vi "Insert_SubPnl.vi"(0 "reference in":refnum<class "GUI.lvclass">, 1 "SubPnl":refnum<vi>, 11 "error in (no error)":errorcluster) -> (4 "reference out":refnum<class "GUI.lvclass">, 14 "dt":u32, 15 "error out":errorcluster)   [LabVIEW 2019, in "GUI.lvclass"]
uses:
  GUI.lvclass
  GUI.lvclass/GUI.ctl
  WindowsState.ctl
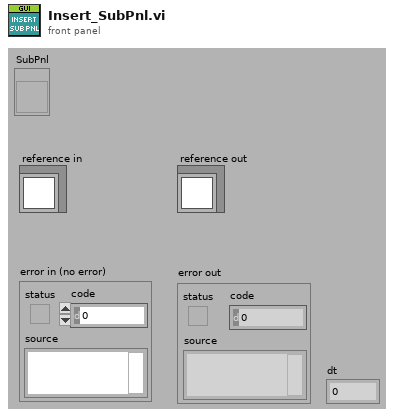
[diagram p1: front panel]
types:
  T1 = typedef "GUI.lvclass/WindowsState.ctl" = enum16{"NotReady", "Ready", "Inserted", "Opened"}
  T2 = typedef "GUI.lvclass/Shered Data.ctl" = cluster{"WindowsState":T1, "UI VI":refnum<vi>, "SubPnl":refnum<vi>}
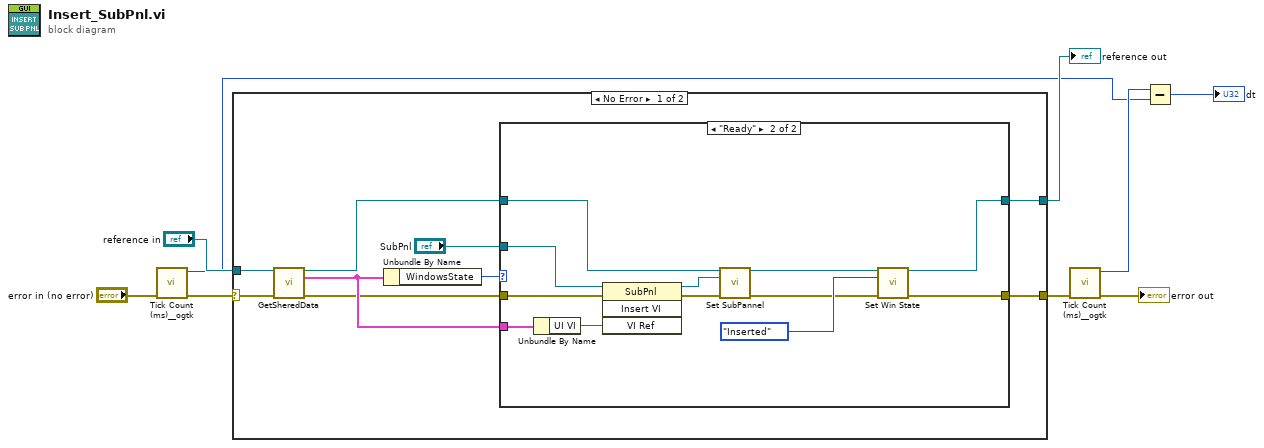
[diagram p0: block diagram]
diagram:
  n1 = call <userlib>:"Tick Count (ms)__ogtk.vi"("error in (no error)"="error in (no error)") -> ("error out"=w6:errorcluster, "millisecond timer value"=w2:u32)  [unwired: 9 in]
  n2 = case shown="No Error" w6 {
    selector: w6 -> [w13 w34]
    tunnel: [w17 w34] -> w5
    tunnel: [w15 w33] -> w8
    tunnel: "reference in" -> [w11 w33]
    frame No Error {
      n3 = call "GetSheredData.vi"("reference in"=w11, "error in (no error)"=w13) -> ("reference out"=w10:refnum<class "GUI.lvclass">, "data"=w14:T2, "error out"=w12:errorcluster)  [unwired: 11 in]
      n4 = Unbundle By Name(w14) -> ("WindowsState"=w16:T1)
      n5 = case shown="\"Ready\"" w16 {
        tunnel: "SubPnl" -> [_ w32]
        tunnel: [w20 w29] -> w17
        tunnel: w12 -> [w20 w26]
        tunnel: w14 -> [_ w31]
        tunnel: w10 -> [w19 w22]
        tunnel: [w19 w28] -> w15
        frame "NotReady", Default {
        }
        frame "Ready" {
          n6 = Unbundle By Name(w31) -> ("UI VI"=w30:refnum<vi>)
          n7 = invoke on="Invoke Node" class="SubPnl" method="Insert VI"(reference=w32, error in=w26, "VI Ref"=w30) -> (reference out=w25:refnum<vi>, error out=w24:errorcluster)  [unwired: 1 in, 2 out]
          n8 = call "Set SubPannel.vi"("reference in"=w22, "SubPnl"=w25, "error in (no error)"=w24) -> ("reference out"=w21:refnum<class "GUI.lvclass">, "error out"=w23:errorcluster)  [unwired: 11 in]
          n9 = call "Set Win State.vi"("reference in"=w21, "WindowsState"=WindowsState."Inserted", "error in (no error)"=w23) -> ("reference out"=w28:refnum<class "GUI.lvclass">, "error out"=w29:errorcluster)  [unwired: 11 in]
        }
      }
    }
    frame Error {
    }
  }
  "reference out" <- w8
  n10 = call <userlib>:"Tick Count (ms)__ogtk.vi"("error in (no error)"=w5) -> ("error out"=→"error out":errorcluster, "millisecond timer value"=w3:u32)  [unwired: 9 in]
  n11 = Subtract(x=w3, y=w2) -> (x-y=→"dt":u32)
